vi "Position.vi"(11 "Square in":refnum<class "Square.lvclass">) -> (2 "Position":T1)   [LabVIEW 2020, in "SquareBattle.lvlib" / "Square.lvclass"]
doc: "Returns the current position of the square. Coordinates run from (0,0) in the bottom left and increase in the NE direction."
uses:
  Square.lvclass
  Position.ctl
  Square.lvclass/Square.ctl
  SquareBattle.lvlib
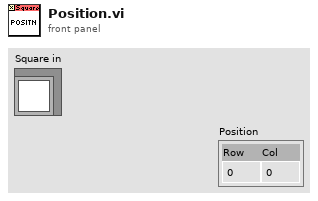
[diagram p1: front panel]
types:
  T1 = typedef "SquareBattle.lvlib/Position.ctl" = cluster{"Row":i32, "Col":i32}
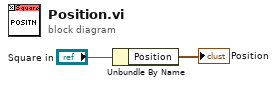
[diagram p0: block diagram]
diagram:
  n1 = Unbundle By Name("Square in") -> ("Position"=→"Position":T1)
